vi "Motion manual controls silver.vi"() -> ()   [LabVIEW 2017]
panel:
  in  "X Home Button 4":bool
  in  "X Jog Neg. 4":bool
  in  "X Jog Pos. 4":bool
  in  "X Home Button 3":bool
  in  "X Jog Neg. 3":bool
  in  "X Jog Pos. 3":bool
  in  "X Home Button 2":bool
  in  "X Jog Neg. 2":bool
  in  "X Jog Pos. 2":bool
  in  "X Home Button":bool
  in  "X Jog Neg.":bool
  in  "X Jog Pos.":bool
  out "Boolean 4":bool
  in  "SetZOrigin 4":bool
  in  "Position,mm 5":sgl caption="R Position, degrees" format="%.4f"
  in  "Set R Position, Deg.":sgl format="%.4f"
  out "Boolean 3":bool
  in  "SetZOrigin 3":bool
  in  "Position,mm 4":sgl caption="Z Position, mm" format="%.4f"
  in  "Set Z Position, mm":sgl format="%.4f"
  out "Boolean 2":bool
  in  "SetZOrigin 2":bool
  in  "Position,mm 3":sgl caption="Y Position, mm" format="%.4f"
  in  "Set Y Position, mm":sgl format="%.4f"
  out "Boolean":bool
  in  "SetZOrigin":bool
  in  "Position,mm":sgl caption="X Position, mm" format="%.4f"
  in  "Set X Position, mm":sgl format="%.4f"
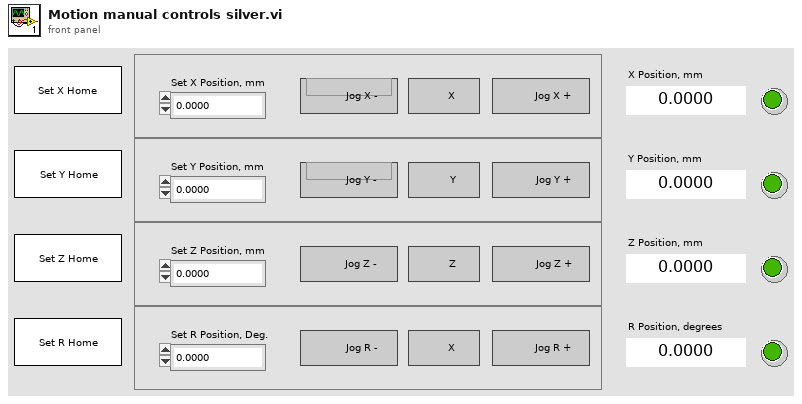
[diagram p1: front panel]
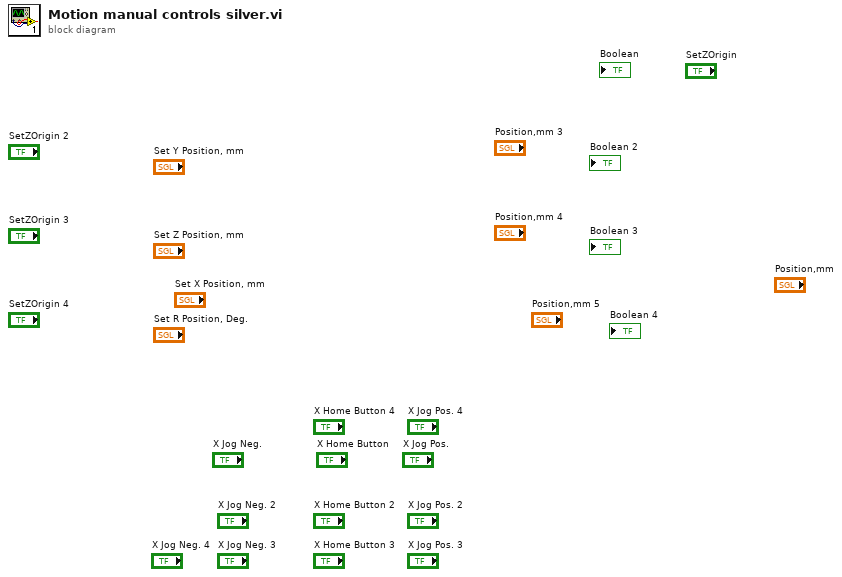
[diagram p0: block diagram]
diagram:
